vi "WPI_CANJaguar_CheckConfig.vi"(11 "CAN Jaguar Ref":T1={"DeviceStatus"={"status"=FALSE, "code"=0, "source"=""}, "Type"=enum."PWM", "PWM"={"PWM Channel"=enum."PWM 1", "DeadBand"={"Name"="", "maxPositivePwm"=0, "minPositivePwm"=0, "centerPwm"=0, "maxNegativePwm"=0, "minNegativePwm"=0, "angularRange"=0}}, "CAN"={"Device Number"=0, "SetOutput VI Ref"=variant(enum8{"Percent VBus", "Current", "Speed", "Position", "Voltage"} enum."Percent VBus"), "GetOutput VI Ref"=variant(refnum<k1> refnum), "Enable VI Ref"=variant(dbl 12.0), "Disable VI Ref"=variant(enum8{"Percent VBus", "Speed", "Position", "Slave", "Unchanged / Invalid", "Voltage Compensation", "Current", "Motion Profile"} enum."Percent VBus"), "Data"=variant}, "Invert"=FALSE}) -> (2 "Warning":bool)   [LabVIEW 2016]
uses:
  <vilib>/Rock Robotics/WPI/MotorControl/WPI_MotorControlDeviceRef.ctl
  <vilib>/Rock Robotics/WPI/MotorControl/WPI_MotorControlType.ctl
  <vilib>/Rock Robotics/SystemInterfaces/DIO/FPGA_DIOPWMChannel.ctl
  <vilib>/Rock Robotics/WPI/PWM/WPI_PWMDeadband.ctl
  <vilib>/Rock Robotics/WPI/ThirdParty/CanMotor/CAN Jaguar/SubVIs/WPI_CANJaguar_ControlMode.ctl
  <vilib>/Rock Robotics/WPI/ThirdParty/CanMotor/CAN Jaguar/SubVIs/WPI_CAN_MotorMessageIDs.ctl
  <vilib>/Rock Robotics/WPI/ThirdParty/CanMotor/CAN Jaguar/SubVIs/WPI_CANJaguar_StatusSelect.ctl
  <vilib>/Rock Robotics/WPI/ThirdParty/CanMotor/CAN Jaguar/SubVIs/WPI_CANJaguar_RefNumData.ctl
panel:
  in  "Force":bool
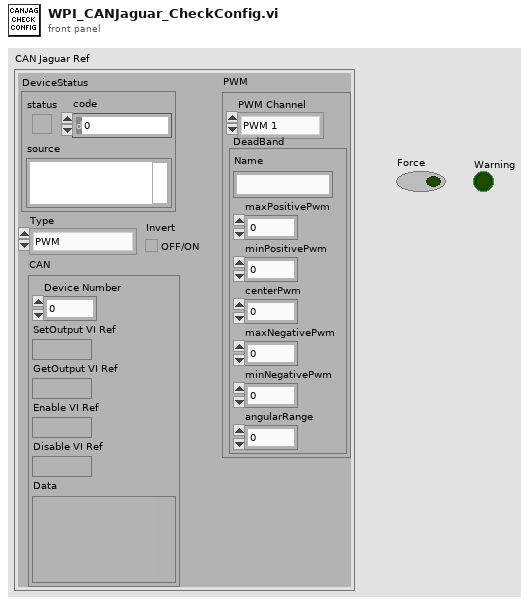
[diagram p1: front panel]
types:
  T1 = typedef "WPI_MotorControlDeviceRef.ctl" = cluster{"DeviceStatus":errorcluster, "Type":T2, "PWM":cluster{"PWM Channel":T3, "DeadBand":T4}, "CAN":cluster{"Device Number":u8, "SetOutput VI Ref":variant, "GetOutput VI Ref":variant, "Enable VI Ref":variant, "Disable VI Ref":variant, "Data":variant}, "Invert":bool}
  T2 = typedef "WPI_MotorControlType.ctl" = enum16{"PWM", "CAN"}
  T3 = typedef "FPGA_DIOPWMChannel.ctl" = enum8{"PWM 0", "PWM 1", "PWM 2", "PWM 3", "PWM 4", "PWM 5", "PWM 6", "PWM 7", "PWM 8", "PWM 9", "PWM MXP 0", "PWM MXP 1", "PWM MXP 2", "PWM MXP 3", "PWM MXP 4", "PWM MXP 5", "PWM MXP 6", "PWM MXP 7", "PWM MXP 8", "PWM MXP 9", "Invalid"}
  T4 = typedef "WPI_PWMDeadband.ctl" = cluster{"Name":string, "maxPositivePwm":i32, "minPositivePwm":i32, "centerPwm":i32, "maxNegativePwm":i32, "minNegativePwm":i32, "angularRange":u16}
  T5 = typedef "WPI_CANJaguar_StatusSelect.ctl" = enum16{"Output Percent VBus", "Output Voltage", "Bus Voltage", "Current", "Temperature", "Position", "Speed", "Limit Switches", "Faults", "Fault Counters", "Power Cycle"}
  T6 = typedef "WPI_CANJaguar_ControlMode.ctl" = enum8{"Percent VBus", "Current", "Speed", "Position", "Voltage"}
  T7 = typedef "WPI_CAN_MotorMessageIDs.ctl" = u32
  T8 = cluster{"CAN.Control Mode":T6, "Squelched Messages":T7[]}[]
  T9 = typedef "WPI_CANJaguar_Status.ctl" = cluster{"Output Percent VBus":dbl, "Output Voltage":dbl, "Bus Voltage":dbl, "Current":dbl, "Temperature":dbl, "Position":dbl, "Speed":dbl, "Limits":cluster{"Forward Limit":bool, "Reverse Limit":bool, "Forward Soft Limit":bool, "Reverse Soft Limit":bool, "Sticky Forward Limit":bool, "Sticky Reverse Limit":bool, "Sticky Forward Soft Limit":bool, "Sticky Reverse Soft Limit":bool}, "Faults":cluster{"Current Fault":bool, "Temperature Fault":bool, "Bus Voltage Fault":bool, "Gate Driver Fault":bool, "Comm Fault":bool}, "Fault Counters":cluster{"Current Faults":u8, "Temperature Faults":u8, "Bus Voltage Faults":u8, "Gate Driver Faults":u8, "Comm Faults":u8, "CAN Status":u8, "CAN RX Errors":u8, "CAN TX Errors":u8}, "Power Cycle":bool}
  T10 = typedef "WPI_CANJaguar_ConfigMessage.ctl" = cluster{"Message ID":u32, "Needs Check":bool, "Data":u8[], "Mode":bool}
  T11 = typedef "WPI_CANJaguar_RefNumData.ctl" = cluster{"CAN.Max Vout":dbl, "Control Mode":T6, "semaphore":T12}
  T12 = typedef "Semaphore RefNum" = refnum<k1>
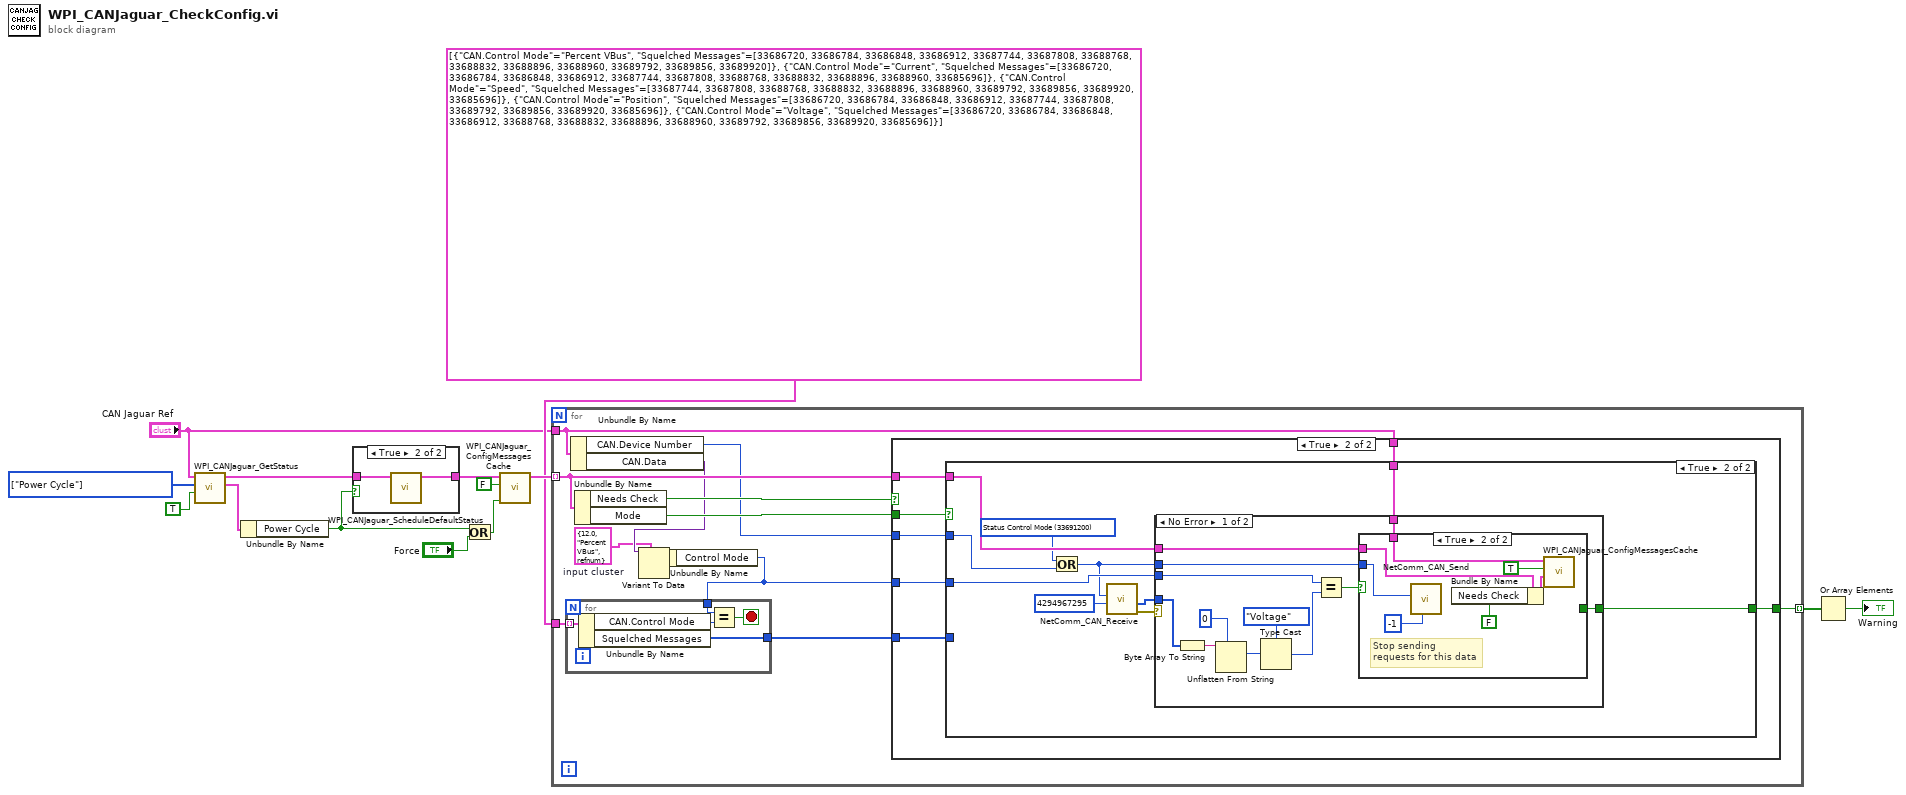
[diagram p0: block diagram]
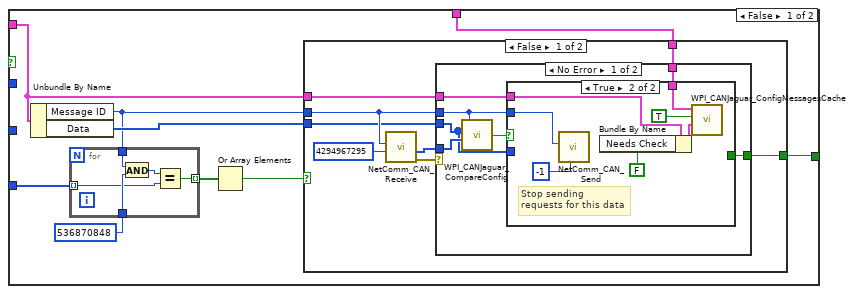
[diagram p4: hidden frame]
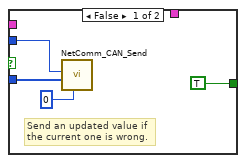
[diagram p5: hidden frame]
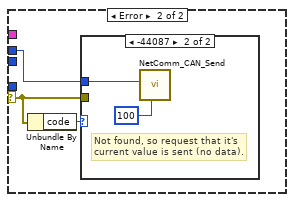
[diagram p6: hidden frame]
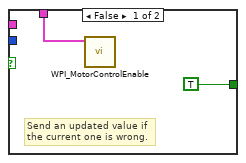
[diagram p9: hidden frame]
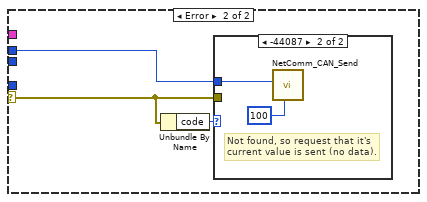
[diagram p10: hidden frame]
diagram:
  w10 = T5[] [enum."Power Cycle"] items=["Output Percent VBus", "Output Voltage", "Bus Voltage", "Current", "Temperature", "Position", "Speed", "Limit Switches", "Faults", "Fault Counters", "Power Cycle"] ("Status Select")
  n1 = call <vilib>:"WPI_CANJaguar_GetStatus.vi"("Force On-Demand"=TRUE, "Status Select"=w10, "CAN Jaguar Ref"="CAN Jaguar Ref") -> ("Status"=w9:T9, "CAN Jaguar Ref"=w3:T1)  [unwired: 6 in, 1 out]
  n2 = Unbundle By Name(w9) -> ("Power Cycle"=w1:bool)
  n3 = case shown="True" w1 {
    tunnel: w3 -> [w15 w17]
    tunnel: [w15 w16] -> w2
    frame False {
    }
    frame True {
      n4 = call <vilib>:"WPI_CANJaguar_ScheduleDefaultStatus.vi"("CAN Jaguar Ref Out in"=w17) -> ("CAN Jaguar Ref Out out"=w16:T1)  [unwired: 9 in, 1 out]
    }
  }
  n5 = Or(x=w1, y="Force") -> (x .or. y?=w6:bool)
  n6 = call <vilib>:"WPI_CANJaguar_ConfigMessagesCache.vi"("Check All"=w6, "Update"=FALSE, "CAN Jaguar Ref"=w2) -> ("Config Message Cache"=w14:T10[])  [unwired: 8 in]
  n7 = for {
    tunnel: w14 -> [w28] mode=indexing
    tunnel: "CAN Jaguar Ref" -> [w27]
    tunnel: [w25] -> w13 mode=indexing
    tunnel: T8 [{"CAN.Control Mode"=enum."Percent VBus", "Squelched Messages"=[33686720, 33686784, 33686848, 33686912, 33687744, 33687808, 33688768, 33688832, 33688896, 33688960, 33689792, 33689856, 33689920]}, {"CAN.Control Mode"=enum."Current", "Squelched Messages"=[33686720, 33686784, 33686848, 33686912, 33687744, 33687808, 33688768, 33688832, 33688896, 33688960, 33685696]}, {"CAN.Control Mode"=enum."Speed", "Squelched Messages"=[33687744, 33687808, 33688768, 33688832, 33688896, 33688960, 33689792, 33689856, 33689920, 33685696]}, {"CAN.Control Mode"=enum."Position", "Squelched Messages"=[33686720, 33686784, 33686848, 33686912, 33687744, 33687808, 33689792, 33689856, 33689920, 33685696]}, {"CAN.Control Mode"=enum."Voltage", "Squelched Messages"=[33686720, 33686784, 33686848, 33686912, 33688768, 33688832, 33688896, 33688960, 33689792, 33689856, 33689920, 33685696]}] -> [w24]
    w20 = T11 {"CAN.Max Vout"=12.0, "Control Mode"=enum."Percent VBus", "semaphore"=refnum}  # input cluster
    n8 = Unbundle By Name(w27) -> ("CAN.Device Number"=w22:u8, "CAN.Data"=w21:variant)
    n9 = Unbundle By Name(w28) -> ("Needs Check"=w29:bool, "Mode"=w26:bool)
    n10 = Variant To Data(type=w20, Variant=w21) -> (data=w19:T11)  [unwired: 1 in, 1 out]
    n11 = Unbundle By Name(w19) -> ("Control Mode"=w18:T6)
    n12 = for {
      tunnel: w24 -> [w34] mode=indexing
      tunnel: w18 -> [w32]
      tunnel: [w30] -> w23
      stop <- w31 stop-if-true
      n13 = Unbundle By Name(w34) -> ("CAN.Control Mode"=w33:T6, "Squelched Messages"=w30:T7[])
      n14 = Equal?(x=w32, y=w33) -> (x = y?=w31:bool)
    }
    n15 = case shown="True" w29 {
      tunnel: w28 -> [_ w40]
      tunnel: w27 -> [_ w41]
      tunnel: w18 -> [_ w38]
      tunnel: w26 -> [_ w39]
      tunnel: [_ w37] -> w25
      tunnel: w23 -> [_ w36]
      tunnel: w22 -> [_ w35]
      frame False {
      }
      frame True {
        n16 = case shown="True" w39 {
          tunnel: w41 -> [w49 w94]
          tunnel: w40 -> [w48 w93]
          tunnel: w38 -> [_ w92]
          tunnel: [w47 w91] -> w37
          tunnel: w36 -> [w46 _]
          tunnel: w35 -> [_ w90]
          frame False {
            n17 = Unbundle By Name(w48) -> ("Message ID"=w45:u32, "Data"=w50:u8[])
            n18 = for {
              tunnel: w46 -> [w52] mode=indexing
              tunnel: w45 -> [w55]
              tunnel: u32 536870848 ("Message ID Mask") -> [w54]
              tunnel: [w51] -> w43 mode=indexing
              n19 = And(x=w55, y=w54) -> (x .and. y?=w53:u32)
              n20 = Equal?(x=w53, y=w52) -> (x = y?=w51:bool)
            }
            n21 = Or Array Elements(Boolean array=w43) -> (logical OR=w42:bool)
            n22 = case shown="False" w42 {
              tunnel: w45 -> [w61 _]
              tunnel: w50 -> [w59 _]
              tunnel: w49 -> [w58 _]
              tunnel: w48 -> [w57 _]
              tunnel: [w56 _] -> w47
              frame False {
                n23 = call <vilib>:"NetComm_CAN_Receive.vi"("Message ID Mask"=u32 4294967295, "Message ID"=w61) -> ("error out"=w62:errorcluster, "Data"=w60:u8[])  [unwired: 6 in, 2 out]
                n24 = case shown="No Error" w62 {
                  selector: w62 -> [_ w83]
                  tunnel: w61 -> [w66 w82]
                  tunnel: w60 -> [w70 _]
                  tunnel: w59 -> [w64 _]
                  tunnel: w58 -> [w69 _]
                  tunnel: w57 -> [w68 _]
                  tunnel: [w67 _] -> w56
                  frame No Error {
                    n25 = call <vilib>:"WPI_CANJaguar_CompareConfig.vi"("Received Data"=w70, "Expected Data"=w64, "Message ID"=w66) -> ("Equivalent"=w65:bool)  [unwired: 3 in]
                    n26 = case shown="True" w65 {
                      tunnel: w66 -> [w74 w81]
                      tunnel: w64 -> [w73 _]
                      tunnel: w69 -> [_ w79]
                      tunnel: w68 -> [_ w77]
                      tunnel: [TRUE _] -> w67
                      frame False {
                        # "Send an updated value if the current one is wrong."
                        n27 = call <vilib>:"NetComm_CAN_Send.vi"("Period (ms)"=0, "Data"=w73, "Message ID"=w74) -> ()  [unwired: 8 in, 1 out]
                      }
                      frame True {
                        # "Stop sending requests for this data"
                        n28 = call <vilib>:"NetComm_CAN_Send.vi"("Period (ms)"=-1, "Message ID"=w81) -> ()  [unwired: 9 in, 1 out]
                        n29 = Bundle By Name(cluster=w77, "Needs Check"=FALSE) -> (w76:T10)
                        n30 = call <vilib>:"WPI_CANJaguar_ConfigMessagesCache.vi"("Config Message"=w76, "Update"=TRUE, "CAN Jaguar Ref"=w79) -> ()  [unwired: 8 in, 1 out]
                      }
                    }
                  }
                  frame Error {
                    n31 = Unbundle By Name(w83) -> ("code"=w84:i32)
                    n32 = case shown="-44087" w84 {
                      tunnel: w83 -> [_ _]
                      tunnel: w82 -> [_ w85]
                      frame 0, Default {
                      }
                      frame -44087 {
                        # "Not found, so request that it's current value is sent (no data)."
                        n33 = call <vilib>:"NetComm_CAN_Send.vi"("Period (ms)"=100, "Message ID"=w85) -> ()  [unwired: 9 in, 1 out]
                      }
                    }
                  }
                }
              }
              frame True {
              }
            }
          }
          frame True {
            w89 = T7 33691200 items=["Volt Enable"=33685504, "Volt Disable"=33685568, "Volt Set"=33685632, "Volt Set Ramp"=33685696, "Speed Enable"=33686528, "Speed Disable"=33686592, "Speed Set"=33686656, "Speed P"=33686720, "Speed I"=33686784, "Speed D"=33686848, "Speed Ref"=33686912, "Volt Comp Enable"=33687552, "Volt Comp Disable"=33687616, "Volt Comp Set"=33687680, "Volt Comp In Ramp"=33687744, "Volt Comp Comp Ramp"=33687808, "Position Enable"=33688576, "Position Disable"=33688640, "Position Set"=33688704, "Position P"=33688768, "Position I"=33688832, "Position D"=33688896, "Position Ref"=33688960, "Current Enable"=33689600, "Current Disable"=33689664, "Current Set"=33689728, "Current P"=33689792, "Current I"=33689856, "Current D"=33689920, "Status Percent VBus"=33690624, "Status VBus"=33690688, "Status Current"=33690752, "Status Temp"=33690816, "Status Position"=33690880, "Status Speed"=33690944, "Status Limit"=33691008, "Status Fault"=33691072, "Status Power"=33691136, "Status Control Mode"=33691200, "Status VOut"=33691264, "Config Num Brushes"=33692672, "Config Encoder Lines"=33692736, "Config Pot Turns"=33692800, "Config Brake Coast"=33692864, "Config Limit Mode"=33692928, "Config Limit Fwd"=33692992, "Config Limit Rev"=33693056, "Config Max VOut"=33693120, "Config Fault Time"=33693184, "Motor Ack"=33693696] ("CAN Motor Message IDs")
            n34 = Or(x=w89, y=w90) -> (x .or. y?=w88:T7)
            n35 = call <vilib>:"NetComm_CAN_Receive.vi"("Message ID Mask"=u32 4294967295, "Message ID"=w88) -> ("error out"=w95:errorcluster, "Data"=w87:u8[])  [unwired: 6 in, 2 out]
            n36 = case shown="No Error" w95 {
              selector: w95 -> [_ w119]
              tunnel: w88 -> [w107 w118]
              tunnel: w92 -> [w106 _]
              tunnel: w94 -> [w105 _]
              tunnel: w93 -> [w104 _]
              tunnel: [w103 _] -> w91
              tunnel: w87 -> [w97 _]
              frame No Error {
                n37 = Byte Array To String(unsigned byte array=w97) -> (string=w100:string)
                n38 = Unflatten From String(type=u8 0, binary string=w100) -> (value=w99:u8)  [unwired: 1 in, 4 out]
                n39 = Type Cast(type=WPI_CANJaguar_ControlMode."Voltage" ("Control Mode"), x=w99) -> (*(type *) &x=w98:T6)
                n40 = Equal?(x=w106, y=w98) -> (x = y?=w108:bool)
                n41 = case shown="True" w108 {
                  tunnel: w107 -> [_ w117]
                  tunnel: w105 -> [w110 w115]
                  tunnel: w104 -> [_ w113]
                  tunnel: [TRUE _] -> w103
                  frame False {
                    # "Send an updated value if the current one is wrong."
                    n42 = call <vilib>:"WPI_MotorControlEnable.vi"("CAN MotorDevRef"=w110) -> ()  [unwired: 9 in, 2 out]
                  }
                  frame True {
                    # "Stop sending requests for this data"
                    n43 = call <vilib>:"NetComm_CAN_Send.vi"("Period (ms)"=-1, "Message ID"=w117) -> ()  [unwired: 9 in, 1 out]
                    n44 = Bundle By Name(cluster=w113, "Needs Check"=FALSE) -> (w112:T10)
                    n45 = call <vilib>:"WPI_CANJaguar_ConfigMessagesCache.vi"("Config Message"=w112, "Update"=TRUE, "CAN Jaguar Ref"=w115) -> ()  [unwired: 8 in, 1 out]
                  }
                }
              }
              frame Error {
                n46 = Unbundle By Name(w119) -> ("code"=w120:i32)
                n47 = case shown="-44087" w120 {
                  tunnel: w119 -> [_ _]
                  tunnel: w118 -> [_ w121]
                  frame 0, Default {
                  }
                  frame -44087 {
                    # "Not found, so request that it's current value is sent (no data)."
                    n48 = call <vilib>:"NetComm_CAN_Send.vi"("Period (ms)"=100, "Message ID"=w121) -> ()  [unwired: 9 in, 1 out]
                  }
                }
              }
            }
          }
        }
      }
    }
  }
  n49 = Or Array Elements(Boolean array=w13) -> (logical OR=→"Warning":bool)
